vi "Mutation v1.vi"(9 "Mutation[%]":dbl=5.0, 11 "Path In":T1={"Distance"=0.0, "Tour"=[1, 14, 13, 12, 7, 6, 15, 5, 11, 9, 10, 16, 3, 2, 4, 8, 1]}) -> (3 "Path Out":T1={"Distance"=0.0, "Tour"=[68, 82, 14, 66, 38, 76, 91, 89, 87, 84, 25, 25, 88]})   [LabVIEW 2015, in "TSP Library.lvlib"]
uses:
  TSP Library.lvlib
  TypeDef/Path.ctl
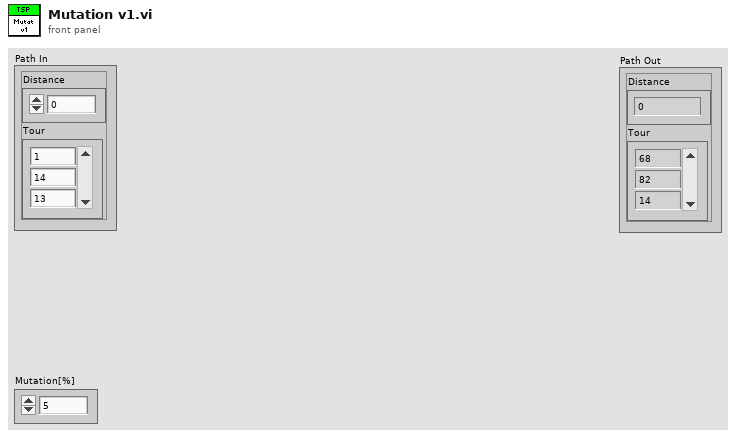
[diagram p1: front panel]
types:
  T1 = typedef "TSP Library.lvlib/Path.ctl" = cluster{"Distance":dbl, "Tour":u16[]}
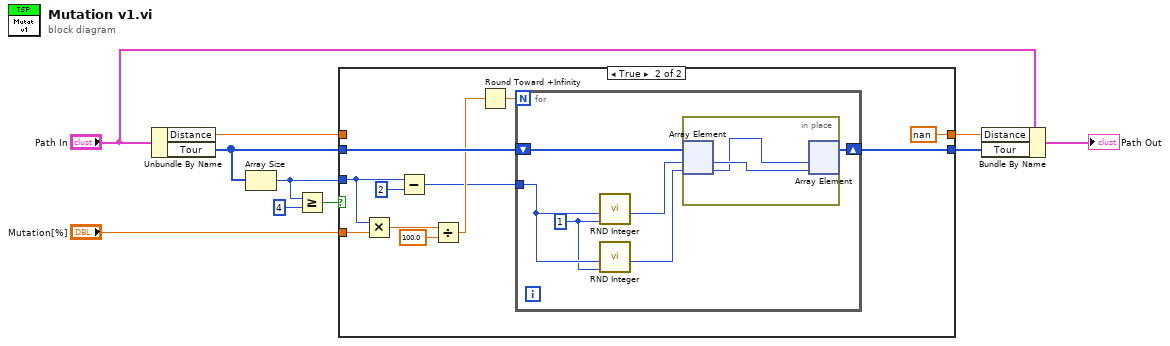
[diagram p0: block diagram]
diagram:
  n1 = Unbundle By Name("Path In") -> ("Distance"=w2:dbl, "Tour"=w7:u16[])
  n2 = Array Size(array=w7) -> (size(s)=w5:i32)
  n3 = Greater Or Equal?(x=w5, y=4) -> (x >= y?=w3:bool)
  n4 = case shown="True" w3 {
    tunnel: [w12 w15] -> w8
    tunnel: w7 -> [w12 w23]
    tunnel: "Mutation[%]" -> [_ w22]
    tunnel: w5 -> [_ w16]
    tunnel: w2 -> [w11 _]
    tunnel: [w11 nan ("Distance")] -> w1
    frame False {
    }
    frame True {
      n5 = Multiply(x=w16, y=w22) -> (x*y=w21:dbl)
      n6 = Subtract(x=w16, y=2) -> (x-y=w18:i32)
      n7 = Divide(x=w21, y=100.0) -> (x/y=w19:dbl)
      n8 = Round Toward +Infinity(x=w19) -> (ceil(x): smallest int >= x=w14:dbl)
      n9 = for {
        N: w14 -> [_]
        tunnel: w18 -> [w27]
        shift-right: [w28] -> w15
        shift-left: w23 -> [w29]
        w24 = 1 ("Min")
        n10 = call "RND Integer.vi"("Min"=w24, "Max"=w27) -> ("RND Integer"=w26:i32)  [unwired: 9 in]
        n11 = call "RND Integer.vi"("Min"=w24, "Max"=w27) -> ("RND Integer"=w25:i32)  [unwired: 9 in]
        n12 = in-place {
          n13 = in-place-array #1(w29, w26, w25) -> (w31:u16, w30:u16)
          n14 = in-place-array #1(w30, w31) -> (w28:u16[])  [unwired: 2 out]
        }
      }
    }
  }
  n15 = Bundle By Name(cluster="Path In", "Distance"=w1, "Tour"=w8) -> (→"Path Out":T1)
